vi "Constant.vi"() -> ()   [LabVIEW 2017]
panel:
  out "power":i8
  out "servo 4":u8
  out "servo 3":u8
  out "servo 2":u8
  out "servo 1":u8
  in  "b_pos":i32
  in  "f_pos":i32
  in  "r_pos":i32
  in  "l_pos":i32
  in  "r_wheel":dbl
  in  "r_car":dbl
  # "= 269.54 mm"
  # "= 101.5 mm"
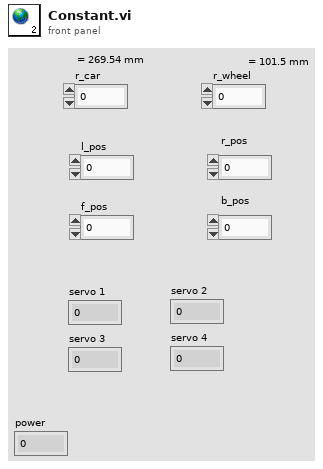
[diagram p1: front panel]
diagram:
